vi "tiffVersion.vi"() -> (3 "tiff_ver":string)   [LabVIEW 2013]
uses:
  imagereconstruction/x64/Release/labviewdll.dll
panel:
  in  "tiff_ver 2":string
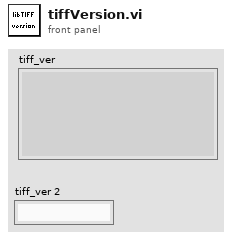
[diagram p1: front panel]
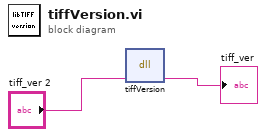
[diagram p0: block diagram]
diagram:
  n1 = dll-call lib="D:/work/uni/FYP/reconrepo/imagereconstruction/x64/Release/labviewdll.dll" fn="tiffVersion"("tiff_ver"="tiff_ver 2") -> ("tiff_ver"=→"tiff_ver":string)  [unwired: 4 in, 2 out]
